vi "RS232_IniByDescription.vi"(11 "Description":string="TTL232RG-3V3_Application") -> (0 "Handle":u32, 1 "COM Port":refnum<visa-resource-name>, 2 "Device Information":T1 {"Type" items=["FT232B-FT245B", "FT8U232AM-FT8U245AM", "FT8U100AX", "UNKNOWN", "FT2232", "FT232R-FT245R", "FT2232H", "FT4232H", "FT232H"]}, 3 "Ok?":bool)   [LabVIEW 2018]
uses:
  <vilib>/Instr/_visa.llb/VISA Configure Serial Port (Instr).vi
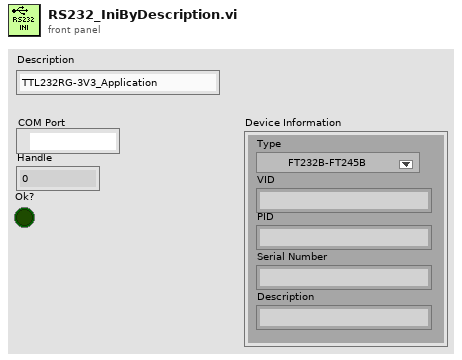
[diagram p1: front panel]
types:
  T1 = cluster{"Type":u32, "VID":string, "PID":string, "Serial Number":string, "Description":string}
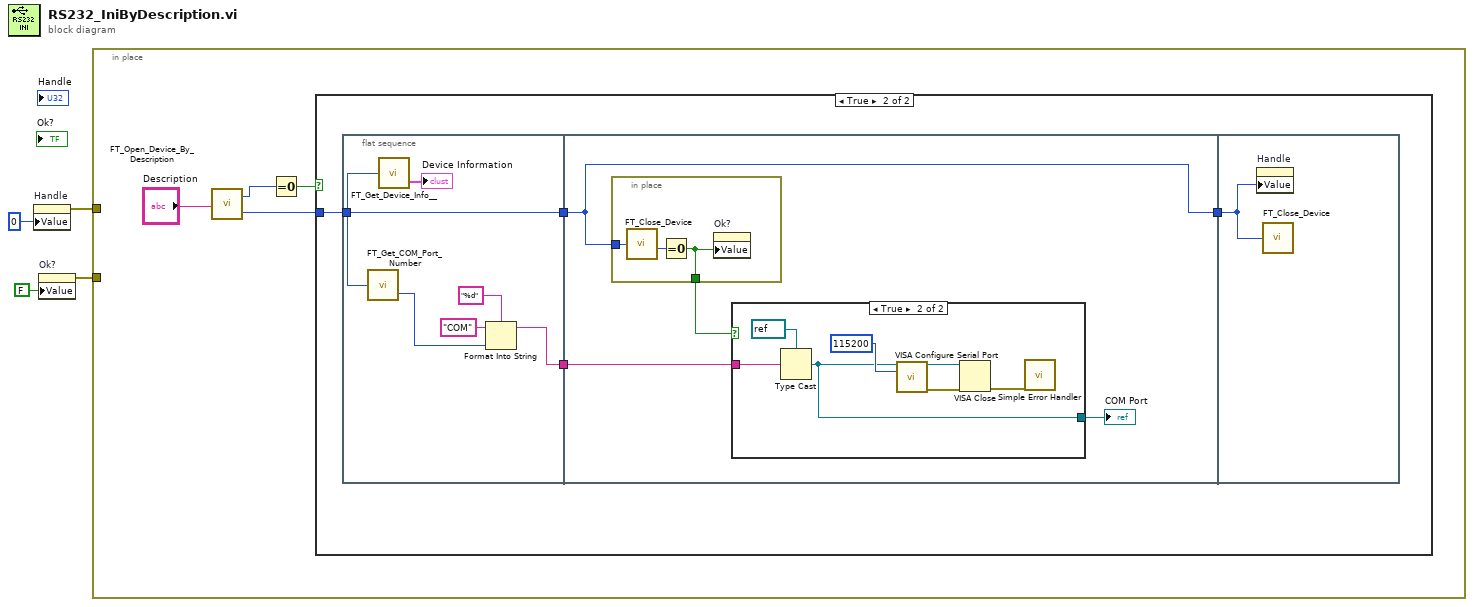
[diagram p0: block diagram]
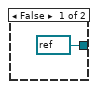
[diagram p3: hidden frame]
diagram:
  n1 = property on="Handle" class="DigNum (strict)"("Value"=u32 0 ("Handle")) -> (error out=w3:errorcluster)  [unwired: 2 in, 1 out]
  n2 = property on="Ok?" class="Bool (strict)"("Value"=FALSE ("Ok?")) -> (error out=w1:errorcluster)  [unwired: 2 in, 1 out]
  n3 = in-place {
    in-place-border: w3 -> [_]
    in-place-border: w1 -> [_]
    n4 = call "FT_Open_Device_By_Description.vi"("Device Description"="Description") -> ("FT_Status"=w7:u32, "Handle"=w5:u32)
    n5 = Equal To 0?(x=w7) -> (x = 0?=w6:bool)
    n6 = case shown="True" w6 {
      tunnel: w5 -> [_ w12]
      frame False {
      }
      frame True {
        n7 = flat-sequence {
          tunnel: w12 -> [w17]
          tunnel: [w17] -> w11
          tunnel: [w13] -> w9
          tunnel: w11 -> [w22]
          tunnel: [w22] -> w10
          tunnel: w9 -> [w20]
          tunnel: w10 -> [w34]
          frame #0 {
            n8 = call "FT_Get_COM_Port_Number.vi"("Handle"=w17) -> ("COM Port Number"=w14:i32)  [unwired: 1 out]
            n9 = call "FT_Get_Device_Info__.vi"("Handle"=w17) -> ("Device Information"=→"Device Information":T1)  [unwired: 1 out]
            n10 = Format Into String(format string="%d", initial string="COM", w14) -> (resulting string=w13:string)  [unwired: 1 in, 1 out]
          }
          frame #1 {
            n11 = in-place {
              in-place-border: w22 -> [w32]
              in-place-border: [w31] -> w21
              n12 = call "FT_Close_Device.vi"("Handle"=w32) -> ("FT_Status"=w33:u32)
              n13 = Equal To 0?(x=w33) -> (x = 0?=w31:bool)
              n14 = property on="Ok?" class="Bool (strict)"("Value"=w31) -> ()  [unwired: 2 in, 2 out]
            }
            n15 = case shown="True" w21 {
              tunnel: w20 -> [_ w28]
              tunnel: [refnum<visa-resource-name> refnum ("VISA resource name") w24] -> w19
              frame False {
              }
              frame True {
                n16 = Type Cast(type=refnum<visa-resource-name> refnum ("VISA resource name"), x=w28) -> (*(type *) &x=w24:refnum<visa-resource-name>)
                n17 = call-poly "VISA Configure Serial Port"("VISA resource name"=w24, "baud rate (9600)"=u32 115200) -> ("VISA resource name out"=w27:refnum<visa-resource-name>, "error out"=w26:errorcluster)  [unwired: 12 in]
                n18 = VISA Close(VISA resource name=w27, error in (no error)=w26) -> (error out=w25:errorcluster)
                n19 = call <vilib>:"Simple Error Handler.vi"("error in (no error)"=w25) -> ()  [unwired: 4 in, 5 out]
              }
            }
            "COM Port" <- w19
          }
          frame #2 {
            n20 = property on="Handle" class="DigNum (strict)"("Value"=w34) -> ()  [unwired: 2 in, 2 out]
            n21 = call "FT_Close_Device.vi"("Handle"=w34) -> ()  [unwired: 1 out]
          }
        }
      }
    }
  }
